vi "CMD_Run Program.vi"(10 "Modules":T1, 11 "Array in":refnum<vi>) -> (3 "output array":string[][](array[string]))   [LabVIEW 2025]
uses:
  Classes/USB IO/Relay Line.ctl
  Libraries/Stepper/Stepper.lvlib
  Libraries/USB IO/USB IO.lvlib
  Libraries/Torque Transducer/Torque Transducer.lvlib
panel:
  out "deleted portion":string[][](array[string])
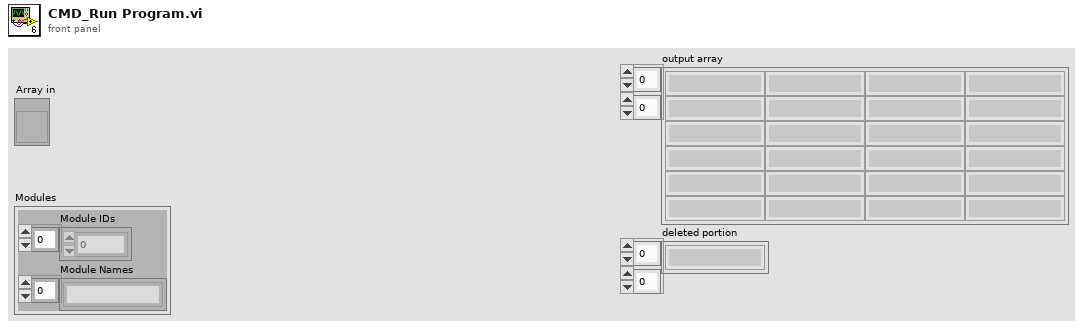
[diagram p1: front panel]
types:
  T1 = cluster{"Module IDs":i32[], "Module Names":string[]}
  T2 = typedef "Relay Line.ctl" = enum16{"+5V", "Brake Relay", "PS Relay"}
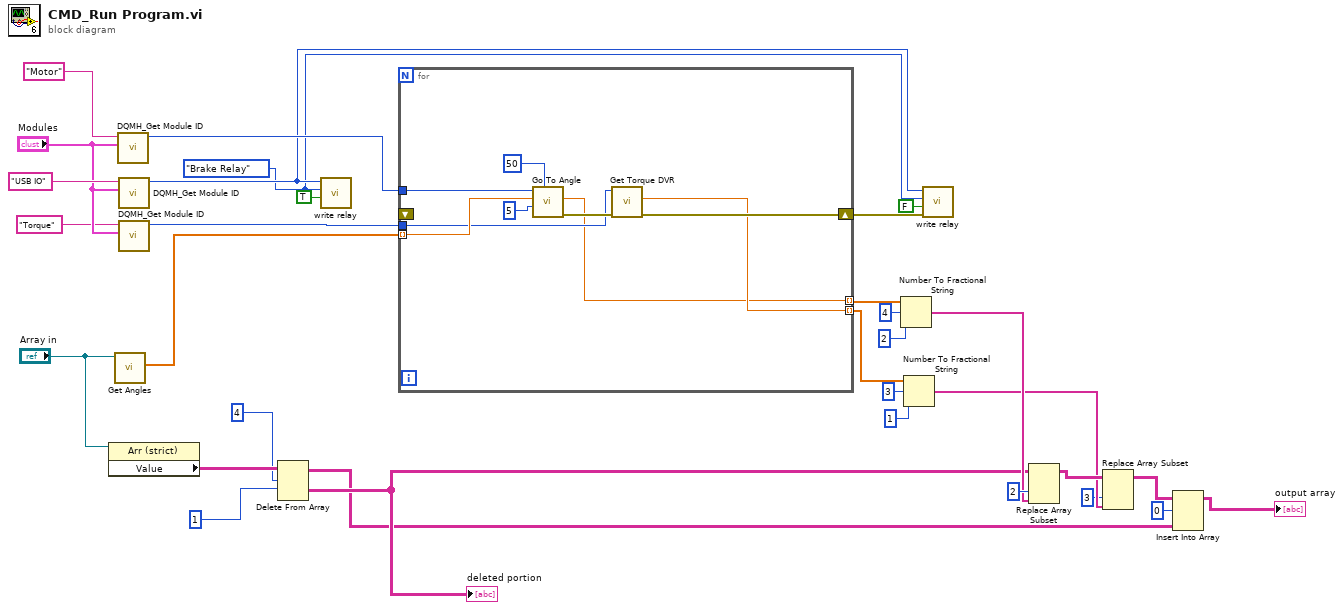
[diagram p0: block diagram]
diagram:
  w24 = Relay_Line."Brake Relay" ("Line Enum")
  n1 = property class="Arr (strict)"(reference="Array in") -> ("Value"=w13:string[][])  [unwired: 1 in, 2 out]
  n2 = call "Get Angles.vi"("Array in"="Array in") -> ("Relative Change"=w32:dbl[])  [unwired: 9 in, 1 out]
  n3 = call "DQMH_Get Module ID.vi"("Modules"="Modules", "Module Name"="Motor") -> ("Module ID out"=w31:i32)  [unwired: 9 in]
  n4 = call "DQMH_Get Module ID.vi"("Modules"="Modules", "Module Name"="USB IO") -> ("Module ID out"=w25:i32)  [unwired: 9 in]
  n5 = call "DQMH_Get Module ID.vi"("Modules"="Modules", "Module Name"="Torque") -> ("Module ID out"=w21:i32)  [unwired: 9 in]
  n6 = Delete From Array(array=w13, length=4, index (row)=1) -> (deleted portion=w8:string[][], array with subset deleted=w3:string[][])  [unwired: 1 in]
  "deleted portion" <- w8
  n7 = call "write relay.vi"("High/Low"=TRUE, "Line Enum"=w24, "Module ID"=w25) -> ()  [unwired: 7 in, 2 out]
  n8 = for {
    tunnel: w32 -> [w40] mode=indexing
    tunnel: w31 -> [w41]
    shift-right: [w35] -> w22
    shift-left: _ -> [_]
    tunnel: w21 -> [w36]
    tunnel: [w34] -> w17 mode=indexing
    tunnel: [w33] -> w20 mode=indexing
    n9 = call "Go To Angle.vi"("Pause Time [ms]"=50, "Velocity [rpm]"=5, "Angle"=w40, "Module ID"=w41) -> ("error out"=w37:errorcluster, "Angle 2"=w33:dbl)  [unwired: 5 in, 1 out]
    n10 = call "Get Torque DVR.vi"("error in"=w37, "Module ID"=w36) -> ("error out"=w35:errorcluster, "Numeric"=w34:dbl)  [unwired: 6 in, 2 out]
  }
  n11 = Number To Fractional String(number=w20, width (-)=i16 4, precision (6)=i16 2) -> (F-format string=w9:string[])  [unwired: 1 in]
  n12 = Number To Fractional String(number=w17, width (-)=i16 3, precision (6)=i16 1) -> (F-format string=w6:string[])  [unwired: 1 in]
  n13 = call "write relay.vi"("error in"=w22, "High/Low"=FALSE, "Line Enum"=w24, "Module ID"=w25) -> ()  [unwired: 6 in, 2 out]
  n14 = Replace Array Subset(array=w8, new element=w9, index (col)=2 ("disabled index (col)")) -> (w7:string[][])  [unwired: 1 in]
  n15 = Replace Array Subset(array=w7, new element=w6, index (col)=3 ("disabled index (col)")) -> (w4:string[][])  [unwired: 1 in]
  n16 = Insert Into Array(array=w4, index (row)=0, new element=w3) -> (→"output array":string[][])  [unwired: 1 in]
